vi "Ultrasonic Loop.vi"   [LabVIEW 2014]
uses:
  <vilib>/Rock Robotics/WPI/Ultrasonic/WPI_UltrasonicRangeUnits.ctl
  Common Code/Ultrasonic Indicators.ctl
  <vilib>/Rock Robotics/WPI/Ultrasonic/WPI_SonarSRF04DigitalRefNum Registry Get.vi
  <vilib>/Rock Robotics/WPI/Ultrasonic/WPI_SonarSRF04DigitalGetRange.vi
  Robot Global Data.vi
types:
  T1 = typedef "Ultrasonic Indicators.ctl" = cluster{"L Dist":dbl, "R Dist":dbl}
  T2 = typedef "WPI_UltrasonicRangeUnits.ctl" = enum16{"inches", "mm"}
  T3 = typedef "WPI_UltrasonicDeviceRef.ctl" = cluster{"DevStatus":errorcluster, "Ping Digital Controller":T4, "Echo Digital Controller":T4, "Ping Channel":T5, "Echo Channel":T5, "CntIndex":T6}
  T4 = typedef "FPGA_TypedefDigitalModule.ctl" = enum16{"Controller 1"}
  T5 = typedef "FPGA_DIOChannel.ctl" = enum8{"DIO 0", "DIO 1", "DIO 2", "DIO 3", "DIO 4", "DIO 5", "DIO 6", "DIO 7", "DIO 8", "DIO 9", "DIO MXP 0", "DIO MXP 1", "DIO MXP 2", "DIO MXP 3", "DIO MXP 4", "DIO MXP 5", "DIO MXP 6", "DIO MXP 7", "DIO MXP 8", "DIO MXP 9", "DIO MXP 10", "DIO MXP 11", "DIO MXP 12", "DIO MXP 13", "DIO MXP 14", "DIO MXP 15", "Invalid"}
  T6 = typedef "FPGA_CounterCtrSystemIndex.ctl" = enum8{"Ctr 0", "Ctr 1", "Ctr 2", "Ctr 3", "Ctr 4", "Ctr 5", "Ctr 6", "Ctr 7", "Invalid"}
  T7 = typedef "WPI_AnalogChannelDevRef.ctl" = cluster{"DevStatus":errorcluster, "Controller":T8, "Analog Channel":T9}
  T8 = typedef "FPGA_TypedefAnalogModule.ctl" = enum16{"Controller 1"}
  T9 = typedef "FPGA_AIChannel.ctl" = enum8{"AI 0", "AI 1", "AI 2", "AI 3", "AI MXP 0", "AI MXP 1", "AI MXP 2", "AI MXP 3", "Invalid"}
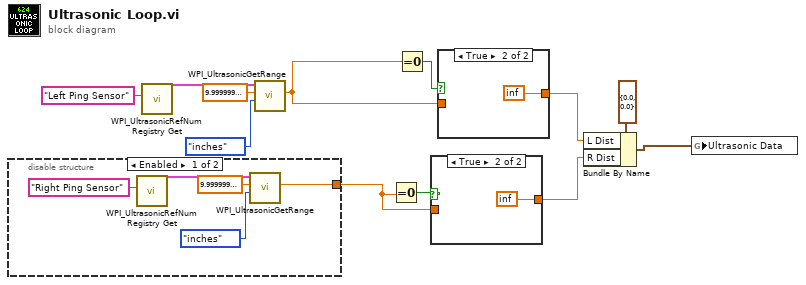
[diagram p0: block diagram]
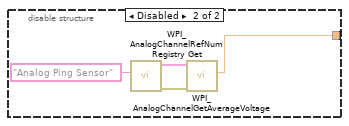
[diagram p4: hidden frame]
diagram:
  n1 = disable-structure shown="Enabled" {
    disable-tunnel: [w13 w18] -> w4
    frame Enabled {
      n2 = call-poly <vilib>:"WPI_UltrasonicRefNum Registry Get.vi"("refnum name"="Right Ping Sensor") -> ("SonarSRF04DevRef"=w16:T3)  [unwired: 9 in, 1 out]
      n3 = call-poly <vilib>:"WPI_UltrasonicGetRange.vi"("Range Units"=WPI_UltrasonicRangeUnits."inches", "ping time (s)"=sgl 1e-05, "SonarSRF04DevRef"=w16) -> ("Distance"=w13:dbl)  [unwired: 6 in, 2 out]
    }
    frame Disabled {
      n4 = call <vilib>:"WPI_AnalogChannelRefNum Registry Get.vi"("refnum name"="Analog Ping Sensor") -> ("error out"=w21:errorcluster, "AIDeviceRef"=w20:T7)  [unwired: 9 in]
      n5 = call <vilib>:"WPI_AnalogChannelGetAverageVoltage.vi"("error in (no error)"=w21, "AIDeviceRef"=w20) -> ("Voltage"=w18:dbl)  [unwired: 7 in, 2 out]
    }
  }
  n6 = call-poly <vilib>:"WPI_UltrasonicRefNum Registry Get.vi"("refnum name"="Left Ping Sensor") -> ("SonarSRF04DevRef"=w12:T3)  [unwired: 9 in, 1 out]
  n7 = call-poly <vilib>:"WPI_UltrasonicGetRange.vi"("Range Units"=WPI_UltrasonicRangeUnits."inches", "ping time (s)"=sgl 1e-05, "SonarSRF04DevRef"=w12) -> ("Distance"=w1:dbl)  [unwired: 6 in, 2 out]
  n8 = Equal To 0?(x=w4) -> (x = 0?=w6:bool)
  n9 = Equal To 0?(x=w1) -> (x = 0?=w3:bool)
  n10 = case shown="True" w6 {
    tunnel: [w22 inf] -> w5
    tunnel: w4 -> [w22 _]
    frame False {
    }
    frame True {
    }
  }
  n11 = case shown="True" w3 {
    tunnel: [w24 inf] -> w2
    tunnel: w1 -> [w24 _]
    frame False {
    }
    frame True {
    }
  }
  n12 = Bundle By Name(cluster=T1 {"L Dist"=0.0, "R Dist"=0.0} ("Ultrasonic Indicators"), "L Dist"=w2, "R Dist"=w5) -> (w7:T1)
  n13 = global write "Robot Global Data.vi" "Ultrasonic Data"(w7) -> ()
